vi "Select Closest Attack Point.vi"(5 "Attack Columns":i32[](array[numeric]), 7 "Attack Rows":i32[](array[numeric]), 10 "Column":i32, 11 "Row":i32) -> (2 "Relative Column Location":i32, 3 "Relative  Row Location":i32)   [LabVIEW 2016, in "AntFarm_MB.lvclass"]
uses:
  AntFarm_MB.lvclass
panel:
  out "distance":dbl
  out "min index(es)":i32
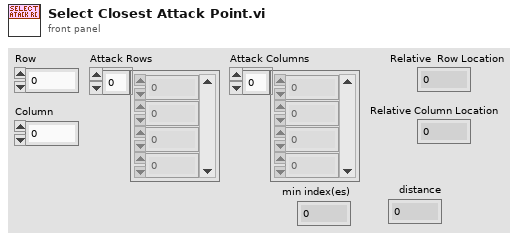
[diagram p1: front panel]
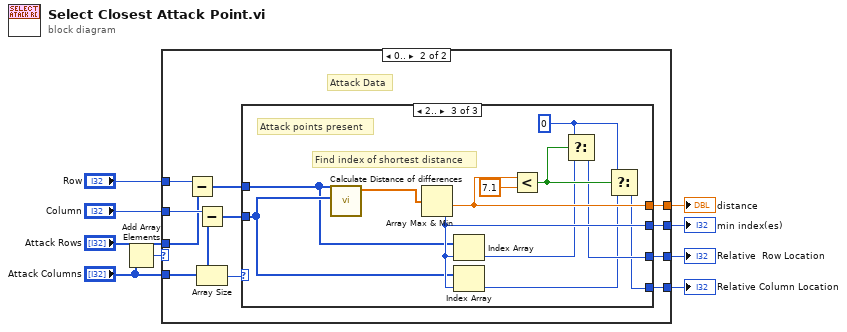
[diagram p0: block diagram]
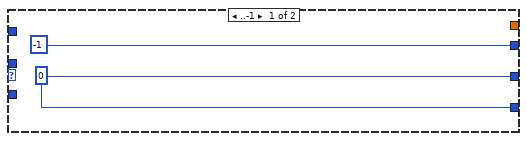
[diagram p2: hidden frame]
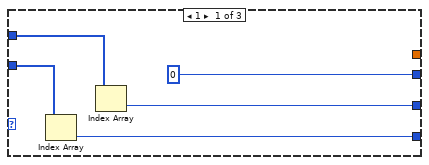
[diagram p3: hidden frame]
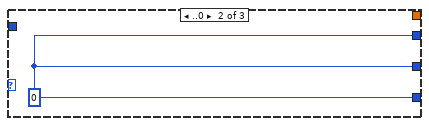
[diagram p4: hidden frame]
diagram:
  n1 = Add Array Elements(numeric array="Attack Columns") -> (sum=w1:i32)
  n2 = case shown="0.." w1 {
    tunnel: "Column" -> [_ w22]
    tunnel: "Row" -> [_ w21]
    tunnel: [w11 w20] -> w7
    tunnel: [w11 w19] -> w6
    tunnel: "Attack Rows" -> [_ w18]
    tunnel: [-1 w17] -> w4
    tunnel: [_ w14] -> w3
    tunnel: "Attack Columns" -> [_ w13]
    frame ..-1 {
      w11 = 0
    }
    frame 0.. {
      # "Attack Data"
      n3 = Subtract(x=w21, y=w18) -> (x-y=w15:i32[])
      n4 = Subtract(x=w22, y=w13) -> (x-y=w16:i32[])
      n5 = Array Size(array=w13) -> (size(s)=w12:i32)
      n6 = case shown="2.." w12 {
        tunnel: [w26 w28 w32] -> w20
        tunnel: [w24 w28 w30] -> w19
        tunnel: [0 w28 w39] -> w17
        tunnel: w16 -> [w25 _ w38]
        tunnel: w15 -> [w27 _ w37]
        tunnel: [_ _ w36] -> w14
        frame 1 {
          n7 = Index Array(array=w25) -> (element=w24:i32)  [unwired: 1 in]
          n8 = Index Array(array=w27) -> (element=w26:i32)  [unwired: 1 in]
        }
        frame ..0 {
          w28 = 0
        }
        frame 2.. {
          w29 = 0 ("t")
          # "Find index of shortest distance"
          # "Attack points present"
          n9 = call "Calculate Distance of differences.vi"("Column Differences"=w38, "Row Differences"=w37) -> ("Array 3"=w40:dbl[])  [unwired: 9 in]
          n10 = Array Max & Min(array=w40) -> (min value=w36:dbl, min index (indices)=w39:i32)  [unwired: 2 out]
          n11 = Index Array(array=w37, index=w39) -> (element=w33:i32)
          n12 = Index Array(array=w38, index=w39) -> (element=w31:i32)
          n13 = Less?(x=w36, y=7.1) -> (x < y?=w34:bool)
          n14 = Select(t=w29, s=w34, f=w33) -> (s? t:f=w32:i32)
          n15 = Select(t=w29, s=w34, f=w31) -> (s? t:f=w30:i32)
        }
      }
    }
  }
  "Relative Column Location" <- w6
  "Relative  Row Location" <- w7
  "min index(es)" <- w4
  "distance" <- w3
